vi "DBsave.vi"(8 "error in (no error)":errorcluster, 11 "FAMM in":refnum<class "FAMM.lvclass">) -> (0 "error out":errorcluster, 3 "FAMM out":refnum<class "FAMM.lvclass">)   [LabVIEW 2014]
doc: "Save unsaved portion of the Historian data to the database."
uses:
  FAMM.lvclass
  DBAL/DBAL.lvclass
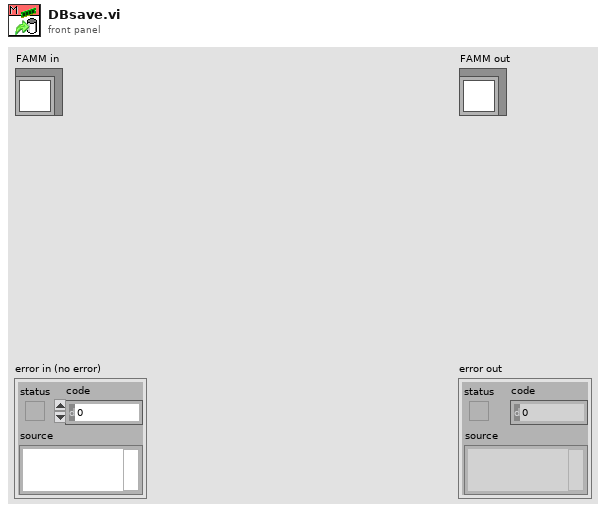
[diagram p1: front panel]
types:
  T1 = cluster{"TableName":string, "Data2save":cluster{"TAGs":string[], "time":dbl[], "TagsData":cluster{"data":dbl[], "max":dbl[], "min":dbl[], "status":u32[]}[]}}[]
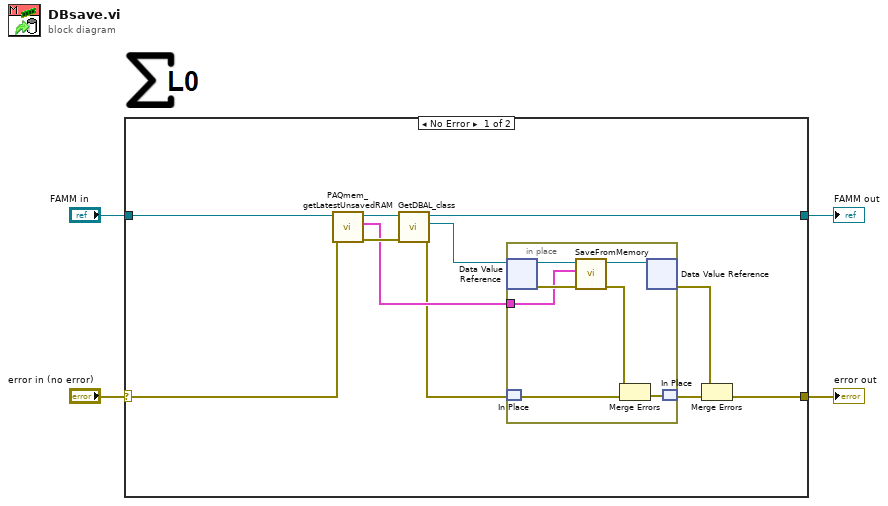
[diagram p0: block diagram]
diagram:
  n1 = case shown="No Error" "error in (no error)" {
    selector: "error in (no error)" -> [w12 w24]
    tunnel: [w13 w24] -> w3
    tunnel: [w14 w23] -> w1
    tunnel: "FAMM in" -> [w15 w23]
    frame No Error {
      n2 = call "PAQmem_getLatestUnsavedRAM.vi"("error in (no error)"=w12, "FAMM in"=w15) -> ("error out"=w10:errorcluster, "Data_2_Save"=w8:T1, "FAMM out"=w11:refnum<class "FAMM.lvclass">)  [unwired: 7 in]
      n3 = call "GetDBAL_class.vi"("error in (no error)"=w10, "FAMM in"=w11) -> ("error out"=w7:errorcluster, "DBAL_class"=w9:refnum<data-value>, "FAMM out"=w14:refnum<class "FAMM.lvclass">)  [unwired: 7 in]
      n4 = in-place {
        in-place-border: w8 -> [w19]
        n5 = in-place-dvr #1(w9) -> (w22:refnum<class "DBAL.lvclass">, w20:errorcluster)
        n6 = in-place-match #2(w7) -> (w18:errorcluster)
        n7 = call-dynamic "SaveFromMemory.vi"("error in (no error)"=w20, "Data_2_Save"=w19, "DBAL in"=w22) -> ("error out"=w17:errorcluster, "DBAL out"=w21:refnum<class "DBAL.lvclass">)  [unwired: 7 in]
        n8 = Merge Errors(w17, w18) -> (w16:errorcluster)
        n9 = in-place-dvr #1(w21) -> (w6:errorcluster)  [unwired: 1 out]
        n10 = in-place-match #2(w16) -> (w5:errorcluster)
      }
      n11 = Merge Errors(w6, w5) -> (w13:errorcluster)
    }
    frame Error {
    }
  }
  "error out" <- w3
  "FAMM out" <- w1
